vi "2_9.vi"() -> ()   [LabVIEW 2015]
panel:
  out "10 elemnets Array":dbl
  out "Last Iteration Number":dbl[](array[numeric])
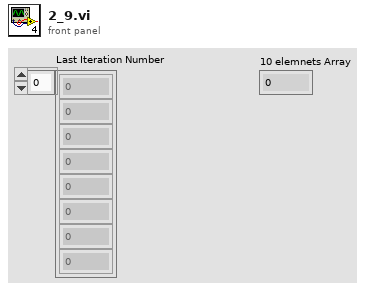
[diagram p1: front panel]
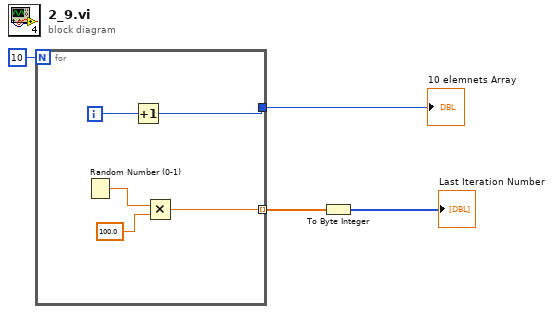
[diagram p0: block diagram]
diagram:
  n1 = for {
    N: 10 -> [_]
    tunnel: [w6] -> w2
    tunnel: [w5] -> w3 mode=indexing
    i -> [w7]
    n2 = Random Number (0-1)() -> (number: 0 to 1=w9:dbl)
    n3 = Increment(x=w7) -> (x+1=w6:i32)
    n4 = Multiply(x=w9, y=100.0) -> (x*y=w5:dbl)
  }
  "10 elemnets Array" <- w2
  n5 = To Byte Integer(number=w3) -> (8bit integer=→"Last Iteration Number":i8[])
